vi "Get (I32 Array).vi"(6 "default timestamp":timestamp, 7 "PV name":string, 8 "error in (no error)":errorcluster, 9 "timeout":dbl[unit]=1.0, 10 "default":i32[](array[numeric]), 11 "Client in":refnum<class "Client.lvclass">) -> (0 "error out":errorcluster, 1 "timed out?":bool, 2 "value":i32[](array[numeric]), 3 "Client out":refnum<class "Client.lvclass">, 4 "timestamp":timestamp)   [LabVIEW 2020, in "PV Access.lvlib" / "PVA Client.lvlib" / "Client.lvclass"]
uses:
  Client.lvclass
  Client.lvclass/Client.ctl
  67d96ea5-d90b-48b4-901c-0faecaf72cae.vi
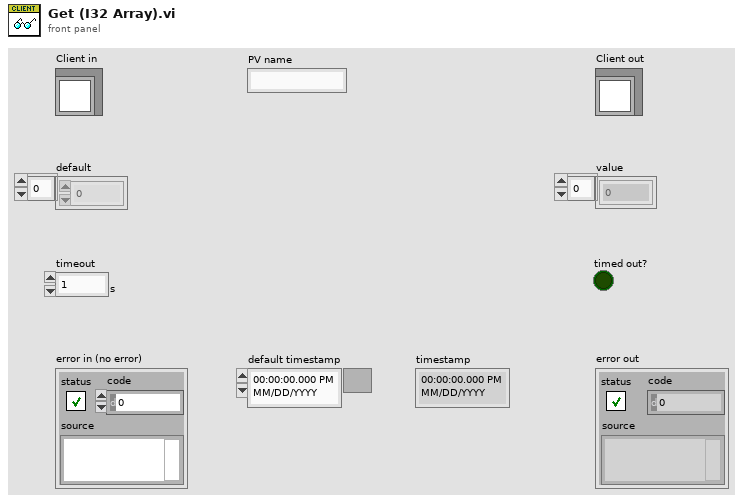
[diagram p1: front panel]
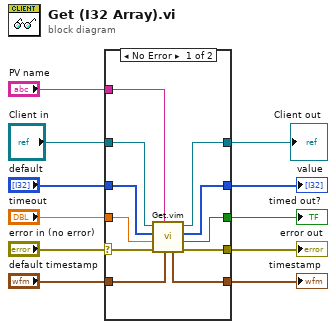
[diagram p0: block diagram]
diagram:
  n1 = case shown="No Error" "error in (no error)" {
    selector: "error in (no error)" -> [w15 w26]
    tunnel: [w14 w26] -> w10
    tunnel: [w16 w25] -> w8
    tunnel: "Client in" -> [w17 w25]
    tunnel: "default" -> [w22 w24]
    tunnel: [w21 w24] -> w6
    tunnel: "timeout" -> [w20 _]
    tunnel: [w19 _] -> w4
    tunnel: "PV name" -> [w18 _]
    tunnel: "default timestamp" -> [w13 w23]
    tunnel: [w12 w23] -> w1
    frame No Error {
      n2 = call "Get.vim"("default timestamp"=w13, "PV name"=w18, "error in"=w15, "timeout"=w20, "default"=w22, "Client in"=w17) -> ("error out"=w14:errorcluster, "timed out?"=w19:bool, "value"=w21:i32[], "Client out"=w16:refnum<class "Client.lvclass">, "timestamp"=w12:timestamp)  [unwired: 1 in]
    }
    frame Error {
    }
  }
  "error out" <- w10
  "Client out" <- w8
  "value" <- w6
  "timed out?" <- w4
  "timestamp" <- w1
